vi "5_VNA_KEYSIGHT_T1_measurements_(Subprog_Rabi).vi"(0 "VNA Power dBm":dbl=5.0 caption="VNA Power, dBm" format="%#.3f", 1 "Center Freq:":dbl=6954420000.0 format="%^#.6e", 2 "Span Freq:":dbl=10000.0 format="%^#.3e", 3 "Bandwidth:":dbl=10.0 caption="Bandwidth (1 to 1e6 Hz):" format="%#.3f", 4 "Sweep Type":i32(ring)=4 caption="Sweep Type:" items=["Lin. Frequency", "Log. Frequency", "Segmented Frequency", "Power", "CW Mode", "Time"], 5 "Points:":i32=4, 6 "File name":string="C:\\ExperimentBlue\\Photon_Source_Dec8'17\\Photon_Source_Dec8'17_Q_osc_05CAL", 7 "Comments":string=" cell Ay\nI=0.0082mA \nf=6.93602GHz\nPulse length sweep 1.5 to 51.5 ns 251 points\nPower  10 to -15 dBm 5 points \nKeysight frequency of pulse generator 10MHz ( 100ns pulse to pulse) \nbandwidth 5Hz\nTransmission Input (VNA):  -chopper1-20-40(4K)\nOut: ~+35dB(4K)+35(RT)", 8 "Dt0 (ns)":dbl=2.0, 9 "Dt1 (ns)":dbl=52.0, 10 "Numeric":u32=251, 11 "save":bool, 12 "Gen Power dBm 2":dbl caption="Gen Power, dBm" format="%#.3f", 13 "Gen Freq:":dbl=10905300000.0 format="%^#.6e") -> (14 "ampl":dbl[](graph)=[-5.350595642994449e-06, -5.748102353209106e-06, -6.142002803244395e-06, -7.127714638954787e-06, -7.280243835339206e-06, -7.58689486701769e-06, -7.235651878545468e-06, -7.886853154559503e-06, -8.111406259558862e-06, -8.24788344289118e-06, -7.998179626156343e-06, -8.358461400348462e-06, -8.104447488221922e-06, -8.498929219058482e-06, -8.536551149518347e-06, -8.1918499290623e-06, -8.209974566852907e-06, -8.195522696041735e-06, -8.220921131396608e-06, -7.921980113678728e-06, -7.674006610614015e-06, -7.494857754863916e-06, -7.402117944366182e-06, -6.798555773457339e-06, -7.21594403785275e-06, -7.021225655989839e-06, -6.167525157252384e-06, -5.991822149553627e-06, -5.853642846886942e-06, -5.251931042948854e-06, -5.243861437520537e-06, -4.8519466417928925e-06, -4.460138825379545e-06, -3.7825817003067637e-06, -3.2926087101259327e-06, -2.9916130301899106e-06, -2.481511216956278e-06, -2.7349177571522887e-06, -1.8771629584080074e-06, -1.5279611602636578e-06, -1.2175324712870859e-06, -5.379010161732367e-07, 6.21079596641039e-08, 8.855542699137692e-08, 4.6134938713748847e-07, 9.043904896088861e-07, 1.3269203407162422e-06, 1.5433369071615743e-06, 1.8643518728822528e-06, 2.399540846909076e-06, 2.143343635907513e-06, 3.011504986716318e-06, 2.7575520675782172e-06, 3.1280499115382554e-06, 3.4887555671048176e-06, 3.906060385361343e-06, 3.6936039009560773e-06, 4.253995143699285e-06, 4.361229116511822e-06, 4.483709631131205e-06, 4.3406083705122e-06, 4.7702748133815476e-06, 5.171184739083401e-06, 4.7876910684863105e-06, 5.051228299635113e-06, 5.085999646325945e-06, 5.146128160049557e-06, 4.943444650962192e-06, 4.87218039779691e-06, 4.565880658446986e-06, 4.918219360661169e-06, 4.184556587460975e-06, 4.655326165448059e-06, 4.499653073253285e-06, 4.171141711140081e-06, 3.84760699034814e-06, 3.771454544221342e-06, 3.763502945730579e-06, 2.8933102385053644e-06, 2.874121037166333e-06, 2.9050245302641997e-06, 2.5922465169969655e-06, 2.1929668321263307e-06, 2.0736858346026565e-06, 1.7167542409879388e-06, 1.4624756374814751e-06, 7.380953093161227e-07, 6.440802060581063e-07, 5.810447483156622e-07, 1.042342834267628e-07, -1.5370875949827212e-07, -5.226669990143761e-07, -7.853622037146126e-07, -1.1198991956007376e-06, -1.5348909698786885e-06, -1.9866505738264095e-06, -1.855540432416092e-06, -2.205690805112681e-06, -2.46238369072671e-06, -2.5284312528128794e-06, -3.0026736226318454e-06, -3.084425941324298e-06, -3.5802571005660857e-06, -3.7021916341473124e-06, -3.686246998313437e-06, -3.4973670040017173e-06, -3.839401415461907e-06, -4.0807350387694905e-06, -4.076152492871189e-06, -4.00435214942263e-06, -4.185059196970542e-06, -4.610368591784209e-06, -4.490104402066208e-06, -4.114603484595135e-06, -4.458382022676233e-06, -4.066545898240292e-06, -3.910781515514827e-06, -4.353571966930759e-06, -3.840349222627992e-06, -3.952571830723173e-06, -3.831163269296667e-06, -3.859261880734265e-06, -3.651557278772088e-06, -3.3495256275273273e-06, -3.446964456088609e-06, -3.3059969837268004e-06, -3.199198999936925e-06, -2.674532879609615e-06, -2.8501009978754155e-06, -2.359338509450027e-06, -2.564694455031713e-06, -2.4649946226418255e-06, -1.9019816477339193e-06, -2.14103451412484e-06, -1.5622521800651155e-06, -1.6103490736441017e-06, -1.6571096637107987e-06, -1.1951571394774874e-06, -1.145164489457784e-06, -9.099043580818036e-07, -4.058469613710259e-07, -5.379223795287658e-07, -3.0455108035454254e-07, -2.0577362391804844e-07, 1.5127773167478138e-07, 3.7407837538694356e-07, 3.06401084060326e-07, 5.40101289914219e-07, 4.2760392915397455e-07, 8.288863710959048e-07, 6.351086767608649e-07, 7.104995063400566e-07, 1.0201038023183173e-06, 1.287821618234375e-06, 1.2846170278635327e-06, 1.1899174978680094e-06, 1.5496536889259005e-06, 1.7193417818361922e-06, 1.2724093494398403e-06, 1.5057571260967961e-06, 1.9633712611266674e-06, 1.5103734369859012e-06, 1.6298976390771713e-06, 1.6734024086417776e-06, 1.480321373037441e-06, 1.6955580974808981e-06, 1.634662169180956e-06, 1.5839247566873382e-06, 1.6462490464164148e-06, 1.4869986841858918e-06, 1.1734323663858959e-06, 1.4257581142373965e-06, 9.750721545742635e-07, 9.460953975803934e-07, 8.49423898330315e-07, 9.841615025152353e-07, 3.2011315020952246e-07, 6.019439595661424e-07, 3.982507532640514e-07, 5.402164049428264e-09, 2.1368394520493444e-07, -3.2420262030541264e-09, -2.370501128723403e-08, -3.75823718812285e-07, -5.397894007330705e-07, -6.145908812982271e-07, -7.628222959965569e-07, -1.1389743690415342e-06, -1.3418293747236025e-06, -1.3894015182813746e-06, -1.369024602126956e-06, -1.6103733457839553e-06, -1.764732246556377e-06, -1.770231932596289e-06, -2.033277155533142e-06, -2.006639647333941e-06, -1.9775290240886534e-06, -1.9851460990594205e-06, -2.3815686063244353e-06, -2.5377885322086513e-06, -2.6544240085968345e-06, -2.5942898105313365e-06, -2.5383228035025236e-06, -3.001205584496347e-06, -2.8813012136197362e-06, -2.361626343372336e-06, -2.9243871040307567e-06, -2.813621961195168e-06, -2.776986320895958e-06, -2.75323276355266e-06, -2.9784823709633193e-06, -2.7528085979611205e-06, -2.9853597993678704e-06, -2.6832433377421694e-06, -2.706799818952277e-06, -2.6102525794158282e-06, -2.5532914378345595e-06, -2.4495236345956073e-06, -2.8292968750065475e-06, -2.7355002885087742e-06, -2.578310500211955e-06, -2.295727739465292e-06, -2.2412349949263444e-06, -2.179298746796121e-06, -2.216602865701134e-06, -2.0977130361643503e-06, -2.037876214444623e-06, -2.1244423464850115e-06, -1.7360226820528626e-06, -1.8201646980742221e-06, -1.7183827480948821e-06, -1.7188583854022004e-06, -1.6155918274307621e-06, -1.6261506914361235e-06, -1.5005421118985398e-06, -1.3091014494648334e-06, -1.3107754170960109e-06, -1.1031796702809515e-06, -1.0116501982793125e-06, -1.0896207669475189e-06, -1.2497122128252158e-06, -9.131707017218105e-07, -8.035339078560353e-07, -7.777753410209698e-07, -8.975365659580346e-07, -8.154549675509772e-07, -7.933004440019431e-07, -4.751387692181199e-07, -4.0351462438081864e-07, -7.113754421084194e-07, -4.4958940748074394e-07], 19 "phase":dbl[](graph)=[-7.019170425337506e-06, -7.572992899440578e-06, -8.083594366325997e-06, -8.282980843432597e-06, -9.005763786262833e-06, -9.200682825394324e-06, -9.523038443148835e-06, -9.838679261520156e-06, -1.0108198466696194e-05, -1.0165816092921887e-05, -1.029021063914115e-05, -1.031981514643121e-05, -1.0695643595681759e-05, -1.0575919532129774e-05, -1.088692602024821e-05, -1.0727918834163575e-05, -1.0352908930144622e-05, -1.0479309594302322e-05, -1.026801805892319e-05, -1.0114804808836197e-05, -9.96231437966344e-06, -1.0128693247679621e-05, -9.729141083880677e-06, -9.54572783484764e-06, -9.351148946734611e-06, -8.996363249025308e-06, -8.951605195761658e-06, -8.266448276117444e-06, -8.23883738121367e-06, -7.827569334040163e-06, -7.317791073546687e-06, -6.8893916704837466e-06, -6.896793706800963e-06, -6.259986207624024e-06, -6.152467562969832e-06, -5.733801913265779e-06, -5.14998862399807e-06, -5.054679149907315e-06, -4.6699628910573665e-06, -4.385781835480884e-06, -3.852076304156071e-06, -3.4347103223808517e-06, -3.1505589390690147e-06, -2.882839055473596e-06, -2.4267251319542993e-06, -2.0543377274861996e-06, -1.8744106853318954e-06, -1.8350467883010424e-06, -1.1185632899923803e-06, -1.2640456645840459e-06, -7.661341072662253e-07, -5.049992815031602e-07, -3.6385645785230736e-07, -4.366051165050068e-08, 3.774253407584638e-07, 5.211261182580529e-07, 4.2912330577848934e-07, 8.784667500094656e-07, 7.522494485101561e-07, 8.956429340400973e-07, 9.095790503010903e-07, 1.184701375223085e-06, 9.438186765464707e-07, 1.0257956688519698e-06, 1.3411245447514375e-06, 1.0582824359062215e-06, 1.352960623535182e-06, 1.153802429598727e-06, 9.581724071949793e-07, 7.940060662292581e-07, 7.361063865118922e-07, 9.280784922793828e-07, 6.255717437397834e-07, 2.950829518511e-07, 5.000459566417703e-07, -2.9220700525911525e-07, -1.555246562645607e-07, -7.036747007305166e-07, -9.239828386853333e-07, -8.351137665840724e-07, -1.3118549304635962e-06, -1.7194672636833275e-06, -1.8967983805850963e-06, -2.3815821350581245e-06, -2.2676868240978365e-06, -3.2337324000764056e-06, -3.3083579751291836e-06, -3.5524304280443175e-06, -3.800510512519395e-06, -3.80134156330314e-06, -4.356420959084062e-06, -4.827017278330459e-06, -5.025575205763744e-06, -5.325945721779135e-06, -5.358401494959253e-06, -6.143812811387761e-06, -6.290685405474505e-06, -6.308485922090767e-06, -6.2665590121468995e-06, -6.645629355261917e-06, -6.524124955831212e-06, -6.957865366530314e-06, -6.78449987390195e-06, -7.311455647140974e-06, -7.419965868393774e-06, -7.837340831429174e-06, -7.111336913112609e-06, -7.561965958302607e-06, -7.808766213202034e-06, -7.69942892020481e-06, -7.712463570896944e-06, -7.581047043458965e-06, -8.152239843184361e-06, -7.779721727274591e-06, -7.729709182058286e-06, -7.868625402807083e-06, -7.543547440036491e-06, -7.2425145845045336e-06, -7.3920455179177225e-06, -7.1634891583016724e-06, -7.435683642142976e-06, -7.109604098332056e-06, -7.161242933761969e-06, -6.776788495699293e-06, -7.035438557068119e-06, -6.850255317658593e-06, -6.483218953690084e-06, -6.188151473907055e-06, -6.034766897755617e-06, -6.058859753466095e-06, -5.548203489524894e-06, -5.673710234077589e-06, -5.174108423489088e-06, -5.141609562997473e-06, -5.159966576684383e-06, -4.946431545249652e-06, -4.847265131502354e-06, -4.7356253389807534e-06, -4.414978661770874e-06, -4.251912287145387e-06, -3.852206191368168e-06, -4.0920668311628106e-06, -3.608850192904356e-06, -3.4423123906890396e-06, -3.716679202625528e-06, -3.326873752484971e-06, -3.0694831139044254e-06, -3.3468560332039488e-06, -3.054596163565293e-06, -2.8194069727760507e-06, -2.8818586770285037e-06, -2.564631074619683e-06, -2.6920887421510997e-06, -2.6940328439195582e-06, -2.4095087098885415e-06, -2.3805068849469535e-06, -2.5056550043700554e-06, -2.443875587232469e-06, -2.177272733661084e-06, -2.4558263476137654e-06, -2.4497868480466423e-06, -2.4176401893782895e-06, -2.682157230537996e-06, -2.536869828873023e-06, -2.40958911490452e-06, -2.6013264005086967e-06, -2.5794037696869054e-06, -3.0161366453285154e-06, -2.6545178002379544e-06, -2.945309233837179e-06, -3.0584037062908465e-06, -3.5290661344333785e-06, -3.1222189136315137e-06, -3.4254662750754505e-06, -3.7309258118511934e-06, -3.883167721596692e-06, -3.7888983683842525e-06, -3.7286271776793e-06, -4.267222948328708e-06, -4.215672788632219e-06, -4.799514613296196e-06, -4.049223491620069e-06, -4.806045012628601e-06, -4.765840685649891e-06, -4.712963459496677e-06, -4.8368552825195366e-06, -5.012265887671674e-06, -5.605749834103335e-06, -5.384020710152981e-06, -5.640716835841886e-06, -5.535724994842894e-06, -5.903570922782819e-06, -5.744383543060394e-06, -6.076711542846169e-06, -5.908389880460163e-06, -6.2967959593152045e-06, -6.162372528706328e-06, -6.263441719056573e-06, -6.3702756278871675e-06, -6.32096828212525e-06, -6.562064413628832e-06, -6.547394150402397e-06, -6.580206786566123e-06, -6.6398285980540095e-06, -6.828778737144603e-06, -6.4207348486888804e-06, -6.490270152426092e-06, -6.515018526442873e-06, -6.581525326510018e-06, -6.594809974558302e-06, -6.453879677792429e-06, -6.79197262343223e-06, -6.798417985010019e-06, -6.491771046057693e-06, -6.526720881083747e-06, -6.384674179571448e-06, -6.509471973004111e-06, -6.414986501113162e-06, -6.234956458683882e-06, -6.2904579181122244e-06, -6.238534183466982e-06, -6.273923645494506e-06, -5.890055604140798e-06, -6.004691272210039e-06, -5.961678311905416e-06, -5.60485193545901e-06, -5.890900865779258e-06, -5.728247288061539e-06, -5.71459065668023e-06, -5.6967975297084195e-06, -5.555835969062173e-06, -5.256393819763616e-06, -5.2477131475825445e-06, -5.247593207968748e-06, -5.350767878553597e-06, -5.333628905646037e-06, -5.198694452701602e-06, -4.963535388924356e-06, -5.009527740185149e-06, -4.453745532373432e-06, -4.926283281747601e-06, -4.547008074951009e-06, -4.7042154847076745e-06, -4.747226967083407e-06, -4.635495542970602e-06, -4.49793731149839e-06, -4.559130957204616e-06, -4.701467787526781e-06, -4.702796445599233e-06, -4.415612238517497e-06, -4.52840652087616e-06])   [LabVIEW 2013]
uses:
  <vilib>/Analysis/NI_AALBase.lvlib
  <vilib>/Analysis/baseanly.llb/Mean (DBL).vi
  <instrlib>/Rohde&Schwarz Vector Network Analyzer/Rohde&Schwarz Vector Network Analyzer.lvlib
panel:
  in  "Ring":u16(ring) items=["Pulse Shift Calibration", "T1 measurement"]
  out "Waveform Graph 2":dbl[](graph)=[-2.2221124422202494, -2.2200494150598864, -2.22054687555374, -2.2813692262672824, -2.2506372258925262, -2.26035908210725, -2.2205431360999093, -2.2465225043911956, -2.247034345801779, -2.252410802151737, -2.2315174356881977, -2.251570699160605, -2.219228532735236, -2.247735449942519, -2.2357730706088486, -2.2229454228604424, -2.241261362587479, -2.234506489472927, -2.245923542606182, -2.235213072381829, -2.2271656113017997, -2.2078427166064345, -2.221185880687629, -2.1896695136273903, -2.2280187758346655, -2.233503304957881, -2.1740916174174107, -2.1979972395375613, -2.1885304421115324, -2.1617605168228144, -2.1925704607839447, -2.1843779293512475, -2.1448463827428856, -2.1143332172734173, -2.0621815638276297, -2.0516924087743607, -2.0198170903435035, -2.066754972840862, -1.9529957650207677, -1.9060358490862137, -1.8769318504176142, -1.726141921489059, -1.551085565186052, -1.5400878525067452, -1.3829263568713952, -1.1560929446483101, -0.9547791124266966, -0.8715305192592462, -0.5404006345918181, -0.4848464421487932, -0.34329462610936456, -0.16614419088094917, -0.13119121203076994, -0.013956835064683466, 0.10776426448886352, 0.13263153817421908, 0.11566157655036537, 0.20364145310501736, 0.17080499526778212, 0.19715986817145928, 0.20656216976967054, 0.24342583588988514, 0.18052791711975594, 0.2110657483169402, 0.2595171973551559, 0.20515025024512784, 0.2570904199282286, 0.22929562642177953, 0.1941838278195652, 0.17217803058580022, 0.14856649652833964, 0.21825376571269267, 0.13357745712488828, 0.06548527695229357, 0.11931287033258386, -0.07579962255318175, -0.04121396317718357, -0.18483912418150655, -0.30911453237721853, -0.2827768403838537, -0.4241682085492582, -0.5856762880987345, -0.7131073752889852, -0.8543968263078259, -0.9227979241818781, -1.1460676995353924, -1.3512908802483115, -1.3914377765807178, -1.419085113448628, -1.5433828019515092, -1.6060649622360101, -1.6786556026742614, -1.7258156155951736, -1.7780493664571155, -1.8497720515141458, -1.8835423107580829, -1.8576287081929448, -1.9071492374579924, -1.9452019952135486, -1.9343498475916896, -2.0021344441342155, -1.9880650878931068, -2.0563664069434715, -2.0395149482186863, -2.0318815202783984, -1.990522446503196, -2.0658511419319145, -2.065650386834191, -2.0518862750216837, -2.0503819785658073, -2.067968101516807, -2.1171825838775367, -2.0742394821005004, -2.0572865701670437, -2.0939712129344246, -2.0477974698596264, -2.049076926431744, -2.1120340406068565, -2.049941304549976, -2.074994602403109, -2.0465616437371685, -2.068113242334879, -2.0423369110411205, -2.0298449758096195, -2.0263660817750417, -2.020434841824136, -2.029196992794578, -1.978751479362645, -2.0120232234838236, -1.9421341611880314, -2.003796081836927, -1.9806514965134467, -1.923060086421989, -1.9653715255507558, -1.8647869786316142, -1.8855325996641679, -1.9002055120394206, -1.8180097653312641, -1.824585110222654, -1.7816153777828392, -1.6757635298129716, -1.7015018190888993, -1.6549869043375756, -1.6305030072196787, -1.5301163900716812, -1.4588252225530398, -1.4713041922306656, -1.4107999761308114, -1.431713078921382, -1.284859462699359, -1.3538820510403298, -1.3005366667363418, -1.2085876850018074, -1.1248807725031937, -1.0809857977123978, -1.1072616226786955, -1.0169119447770274, -0.9577046170580744, -1.041922570804954, -1.0207734830165345, -0.8951744503606424, -1.0123908705644693, -1.0247477161996408, -0.9876791829403154, -1.0198950424763618, -0.9931531132853096, -1.0059392786561479, -1.087231587819844, -1.015678698276403, -1.1032602007634085, -1.2044421445787075, -1.1868426866585982, -1.2680927449116148, -1.3013198155159527, -1.3469409737242553, -1.3225798696208182, -1.4865093650461314, -1.4107387915976213, -1.4777380317239253, -1.5695148798317882, -1.5263037183873518, -1.5715969804305876, -1.5757286191468585, -1.649491275031389, -1.6848323318110747, -1.6971831913424815, -1.7218284748673327, -1.7712473782272706, -1.8150448879730567, -1.8123051545733142, -1.8132389806596525, -1.837097021722014, -1.8688546324376627, -1.8542655068601206, -1.9022356789843693, -1.8792980678558984, -1.8813189423639314, -1.8777226273574936, -1.928564052446991, -1.9525842070365895, -1.9551850148775656, -1.94805057408691, -1.9389592497479615, -1.9953125916293035, -1.9700680868198772, -1.9232507592064303, -1.9941326276753457, -1.9784690362549648, -1.9700693755267644, -1.9662843310264109, -2.0031745533339986, -1.9558660968106016, -1.9845704436945957, -1.962740954169606, -1.9639325880875806, -1.9588923567604022, -1.9445973510447443, -1.9355536099748598, -1.9967890317788455, -1.9809929986786614, -1.9627050215137167, -1.9215790726286834, -1.9343903833346052, -1.9189456958370024, -1.926766066796904, -1.9289245120909744, -1.9038463108288426, -1.9259423843913106, -1.8657244955094845, -1.8800516842623896, -1.8707571123101403, -1.8868391186030182, -1.8694538115127195, -1.8712971229669364, -1.8442082768353885, -1.8114813953939026, -1.817783858710915, -1.7894982571991789, -1.7700615920931608, -1.8107359177553446, -1.819237925501068, -1.7689887938445552, -1.7399750440670247, -1.733191361488536, -1.7620522908712142, -1.7501436462206248, -1.7430740255534625, -1.671516149616777, -1.6563898097010057, -1.7305284307855928, -1.6697540708562737]
  out "No of Values":i32
  in  "Boolean":bool
  out "Pow":dbl=34.32006687269598
  out "Waveform Graph":dbl[][](graph)=[[-5.350595642994449e-06, -5.748102353209106e-06, -6.142002803244395e-06, -7.127714638954787e-06, -7.280243835339206e-06, -7.58689486701769e-06, -7.235651878545468e-06, -7.886853154559503e-06, -8.111406259558862e-06, -8.24788344289118e-06, -7.998179626156343e-06, -8.358461400348462e-06, -8.104447488221922e-06, -8.498929219058482e-06, -8.536551149518347e-06, -8.1918499290623e-06, -8.209974566852907e-06, -8.195522696041735e-06, -8.220921131396608e-06, -7.921980113678728e-06, -7.674006610614015e-06, -7.494857754863916e-06, -7.402117944366182e-06, -6.798555773457339e-06, -7.21594403785275e-06, -7.021225655989839e-06, -6.167525157252384e-06, -5.991822149553627e-06, -5.853642846886942e-06, -5.251931042948854e-06, -5.243861437520537e-06, -4.8519466417928925e-06, -4.460138825379545e-06, -3.7825817003067637e-06, -3.2926087101259327e-06, -2.9916130301899106e-06, -2.481511216956278e-06, -2.7349177571522887e-06, -1.8771629584080074e-06, -1.5279611602636578e-06, -1.2175324712870859e-06, -5.379010161732367e-07, 6.21079596641039e-08, 8.855542699137692e-08, 4.6134938713748847e-07, 9.043904896088861e-07, 1.3269203407162422e-06, 1.5433369071615743e-06, 1.8643518728822528e-06, 2.399540846909076e-06, 2.143343635907513e-06, 3.011504986716318e-06, 2.7575520675782172e-06, 3.1280499115382554e-06, 3.4887555671048176e-06, 3.906060385361343e-06, 3.6936039009560773e-06, 4.253995143699285e-06, 4.361229116511822e-06, 4.483709631131205e-06, 4.3406083705122e-06, 4.7702748133815476e-06, 5.171184739083401e-06, 4.7876910684863105e-06, 5.051228299635113e-06, 5.085999646325945e-06, 5.146128160049557e-06, 4.943444650962192e-06, 4.87218039779691e-06, 4.565880658446986e-06, 4.918219360661169e-06, 4.184556587460975e-06, 4.655326165448059e-06, 4.499653073253285e-06, 4.171141711140081e-06, 3.84760699034814e-06, 3.771454544221342e-06, 3.763502945730579e-06, 2.8933102385053644e-06, 2.874121037166333e-06, 2.9050245302641997e-06, 2.5922465169969655e-06, 2.1929668321263307e-06, 2.0736858346026565e-06, 1.7167542409879388e-06, 1.4624756374814751e-06, 7.380953093161227e-07, 6.440802060581063e-07, 5.810447483156622e-07, 1.042342834267628e-07, -1.5370875949827212e-07, -5.226669990143761e-07, -7.853622037146126e-07, -1.1198991956007376e-06, -1.5348909698786885e-06, -1.9866505738264095e-06, -1.855540432416092e-06, -2.205690805112681e-06, -2.46238369072671e-06, -2.5284312528128794e-06, -3.0026736226318454e-06, -3.084425941324298e-06, -3.5802571005660857e-06, -3.7021916341473124e-06, -3.686246998313437e-06, -3.4973670040017173e-06, -3.839401415461907e-06, -4.0807350387694905e-06, -4.076152492871189e-06, -4.00435214942263e-06, -4.185059196970542e-06, -4.610368591784209e-06, -4.490104402066208e-06, -4.114603484595135e-06, -4.458382022676233e-06, -4.066545898240292e-06, -3.910781515514827e-06, -4.353571966930759e-06, -3.840349222627992e-06, -3.952571830723173e-06, -3.831163269296667e-06, -3.859261880734265e-06, -3.651557278772088e-06, -3.3495256275273273e-06, -3.446964456088609e-06, -3.3059969837268004e-06, -3.199198999936925e-06, -2.674532879609615e-06, -2.8501009978754155e-06, -2.359338509450027e-06, -2.564694455031713e-06, -2.4649946226418255e-06, -1.9019816477339193e-06, -2.14103451412484e-06, -1.5622521800651155e-06, -1.6103490736441017e-06, -1.6571096637107987e-06, -1.1951571394774874e-06, -1.145164489457784e-06, -9.099043580818036e-07, -4.058469613710259e-07, -5.379223795287658e-07, -3.0455108035454254e-07, -2.0577362391804844e-07, 1.5127773167478138e-07, 3.7407837538694356e-07, 3.06401084060326e-07, 5.40101289914219e-07, 4.2760392915397455e-07, 8.288863710959048e-07, 6.351086767608649e-07, 7.104995063400566e-07, 1.0201038023183173e-06, 1.287821618234375e-06, 1.2846170278635327e-06, 1.1899174978680094e-06, 1.5496536889259005e-06, 1.7193417818361922e-06, 1.2724093494398403e-06, 1.5057571260967961e-06, 1.9633712611266674e-06, 1.5103734369859012e-06, 1.6298976390771713e-06, 1.6734024086417776e-06, 1.480321373037441e-06, 1.6955580974808981e-06, 1.634662169180956e-06, 1.5839247566873382e-06, 1.6462490464164148e-06, 1.4869986841858918e-06, 1.1734323663858959e-06, 1.4257581142373965e-06, 9.750721545742635e-07, 9.460953975803934e-07, 8.49423898330315e-07, 9.841615025152353e-07, 3.2011315020952246e-07, 6.019439595661424e-07, 3.982507532640514e-07, 5.402164049428264e-09, 2.1368394520493444e-07, -3.2420262030541264e-09, -2.370501128723403e-08, -3.75823718812285e-07, -5.397894007330705e-07, -6.145908812982271e-07, -7.628222959965569e-07, -1.1389743690415342e-06, -1.3418293747236025e-06, -1.3894015182813746e-06, -1.369024602126956e-06, -1.6103733457839553e-06, -1.764732246556377e-06, -1.770231932596289e-06, -2.033277155533142e-06, -2.006639647333941e-06, -1.9775290240886534e-06, -1.9851460990594205e-06, -2.3815686063244353e-06, -2.5377885322086513e-06, -2.6544240085968345e-06, -2.5942898105313365e-06, -2.5383228035025236e-06, -3.001205584496347e-06, -2.8813012136197362e-06, -2.361626343372336e-06, -2.9243871040307567e-06, -2.813621961195168e-06, -2.776986320895958e-06, -2.75323276355266e-06, -2.9784823709633193e-06, -2.7528085979611205e-06, -2.9853597993678704e-06, -2.6832433377421694e-06, -2.706799818952277e-06, -2.6102525794158282e-06, -2.5532914378345595e-06, -2.4495236345956073e-06, -2.8292968750065475e-06, -2.7355002885087742e-06, -2.578310500211955e-06, -2.295727739465292e-06, -2.2412349949263444e-06, -2.179298746796121e-06, -2.216602865701134e-06, -2.0977130361643503e-06, -2.037876214444623e-06, -2.1244423464850115e-06, -1.7360226820528626e-06, -1.8201646980742221e-06, -1.7183827480948821e-06, -1.7188583854022004e-06, -1.6155918274307621e-06, -1.6261506914361235e-06, -1.5005421118985398e-06, -1.3091014494648334e-06, -1.3107754170960109e-06, -1.1031796702809515e-06, -1.0116501982793125e-06, -1.0896207669475189e-06, -1.2497122128252158e-06, -9.131707017218105e-07, -8.035339078560353e-07, -7.777753410209698e-07, -8.975365659580346e-07, -8.154549675509772e-07, -7.933004440019431e-07, -4.751387692181199e-07, -4.0351462438081864e-07, -7.113754421084194e-07, -4.4958940748074394e-07], [-7.019170425337506e-06, -7.572992899440578e-06, -8.083594366325997e-06, -8.282980843432597e-06, -9.005763786262833e-06, -9.200682825394324e-06, -9.523038443148835e-06, -9.838679261520156e-06, -1.0108198466696194e-05, -1.0165816092921887e-05, -1.029021063914115e-05, -1.031981514643121e-05, -1.0695643595681759e-05, -1.0575919532129774e-05, -1.088692602024821e-05, -1.0727918834163575e-05, -1.0352908930144622e-05, -1.0479309594302322e-05, -1.026801805892319e-05, -1.0114804808836197e-05, -9.96231437966344e-06, -1.0128693247679621e-05, -9.729141083880677e-06, -9.54572783484764e-06, -9.351148946734611e-06, -8.996363249025308e-06, -8.951605195761658e-06, -8.266448276117444e-06, -8.23883738121367e-06, -7.827569334040163e-06, -7.317791073546687e-06, -6.8893916704837466e-06, -6.896793706800963e-06, -6.259986207624024e-06, -6.152467562969832e-06, -5.733801913265779e-06, -5.14998862399807e-06, -5.054679149907315e-06, -4.6699628910573665e-06, -4.385781835480884e-06, -3.852076304156071e-06, -3.4347103223808517e-06, -3.1505589390690147e-06, -2.882839055473596e-06, -2.4267251319542993e-06, -2.0543377274861996e-06, -1.8744106853318954e-06, -1.8350467883010424e-06, -1.1185632899923803e-06, -1.2640456645840459e-06, -7.661341072662253e-07, -5.049992815031602e-07, -3.6385645785230736e-07, -4.366051165050068e-08, 3.774253407584638e-07, 5.211261182580529e-07, 4.2912330577848934e-07, 8.784667500094656e-07, 7.522494485101561e-07, 8.956429340400973e-07, 9.095790503010903e-07, 1.184701375223085e-06, 9.438186765464707e-07, 1.0257956688519698e-06, 1.3411245447514375e-06, 1.0582824359062215e-06, 1.352960623535182e-06, 1.153802429598727e-06, 9.581724071949793e-07, 7.940060662292581e-07, 7.361063865118922e-07, 9.280784922793828e-07, 6.255717437397834e-07, 2.950829518511e-07, 5.000459566417703e-07, -2.9220700525911525e-07, -1.555246562645607e-07, -7.036747007305166e-07, -9.239828386853333e-07, -8.351137665840724e-07, -1.3118549304635962e-06, -1.7194672636833275e-06, -1.8967983805850963e-06, -2.3815821350581245e-06, -2.2676868240978365e-06, -3.2337324000764056e-06, -3.3083579751291836e-06, -3.5524304280443175e-06, -3.800510512519395e-06, -3.80134156330314e-06, -4.356420959084062e-06, -4.827017278330459e-06, -5.025575205763744e-06, -5.325945721779135e-06, -5.358401494959253e-06, -6.143812811387761e-06, -6.290685405474505e-06, -6.308485922090767e-06, -6.2665590121468995e-06, -6.645629355261917e-06, -6.524124955831212e-06, -6.957865366530314e-06, -6.78449987390195e-06, -7.311455647140974e-06, -7.419965868393774e-06, -7.837340831429174e-06, -7.111336913112609e-06, -7.561965958302607e-06, -7.808766213202034e-06, -7.69942892020481e-06, -7.712463570896944e-06, -7.581047043458965e-06, -8.152239843184361e-06, -7.779721727274591e-06, -7.729709182058286e-06, -7.868625402807083e-06, -7.543547440036491e-06, -7.2425145845045336e-06, -7.3920455179177225e-06, -7.1634891583016724e-06, -7.435683642142976e-06, -7.109604098332056e-06, -7.161242933761969e-06, -6.776788495699293e-06, -7.035438557068119e-06, -6.850255317658593e-06, -6.483218953690084e-06, -6.188151473907055e-06, -6.034766897755617e-06, -6.058859753466095e-06, -5.548203489524894e-06, -5.673710234077589e-06, -5.174108423489088e-06, -5.141609562997473e-06, -5.159966576684383e-06, -4.946431545249652e-06, -4.847265131502354e-06, -4.7356253389807534e-06, -4.414978661770874e-06, -4.251912287145387e-06, -3.852206191368168e-06, -4.0920668311628106e-06, -3.608850192904356e-06, -3.4423123906890396e-06, -3.716679202625528e-06, -3.326873752484971e-06, -3.0694831139044254e-06, -3.3468560332039488e-06, -3.054596163565293e-06, -2.8194069727760507e-06, -2.8818586770285037e-06, -2.564631074619683e-06, -2.6920887421510997e-06, -2.6940328439195582e-06, -2.4095087098885415e-06, -2.3805068849469535e-06, -2.5056550043700554e-06, -2.443875587232469e-06, -2.177272733661084e-06, -2.4558263476137654e-06, -2.4497868480466423e-06, -2.4176401893782895e-06, -2.682157230537996e-06, -2.536869828873023e-06, -2.40958911490452e-06, -2.6013264005086967e-06, -2.5794037696869054e-06, -3.0161366453285154e-06, -2.6545178002379544e-06, -2.945309233837179e-06, -3.0584037062908465e-06, -3.5290661344333785e-06, -3.1222189136315137e-06, -3.4254662750754505e-06, -3.7309258118511934e-06, -3.883167721596692e-06, -3.7888983683842525e-06, -3.7286271776793e-06, -4.267222948328708e-06, -4.215672788632219e-06, -4.799514613296196e-06, -4.049223491620069e-06, -4.806045012628601e-06, -4.765840685649891e-06, -4.712963459496677e-06, -4.8368552825195366e-06, -5.012265887671674e-06, -5.605749834103335e-06, -5.384020710152981e-06, -5.640716835841886e-06, -5.535724994842894e-06, -5.903570922782819e-06, -5.744383543060394e-06, -6.076711542846169e-06, -5.908389880460163e-06, -6.2967959593152045e-06, -6.162372528706328e-06, -6.263441719056573e-06, -6.3702756278871675e-06, -6.32096828212525e-06, -6.562064413628832e-06, -6.547394150402397e-06, -6.580206786566123e-06, -6.6398285980540095e-06, -6.828778737144603e-06, -6.4207348486888804e-06, -6.490270152426092e-06, -6.515018526442873e-06, -6.581525326510018e-06, -6.594809974558302e-06, -6.453879677792429e-06, -6.79197262343223e-06, -6.798417985010019e-06, -6.491771046057693e-06, -6.526720881083747e-06, -6.384674179571448e-06, -6.509471973004111e-06, -6.414986501113162e-06, -6.234956458683882e-06, -6.2904579181122244e-06, -6.238534183466982e-06, -6.273923645494506e-06, -5.890055604140798e-06, -6.004691272210039e-06, -5.961678311905416e-06, -5.60485193545901e-06, -5.890900865779258e-06, -5.728247288061539e-06, -5.71459065668023e-06, -5.6967975297084195e-06, -5.555835969062173e-06, -5.256393819763616e-06, -5.2477131475825445e-06, -5.247593207968748e-06, -5.350767878553597e-06, -5.333628905646037e-06, -5.198694452701602e-06, -4.963535388924356e-06, -5.009527740185149e-06, -4.453745532373432e-06, -4.926283281747601e-06, -4.547008074951009e-06, -4.7042154847076745e-06, -4.747226967083407e-06, -4.635495542970602e-06, -4.49793731149839e-06, -4.559130957204616e-06, -4.701467787526781e-06, -4.702796445599233e-06, -4.415612238517497e-06, -4.52840652087616e-06], [8.825963244584914e-06, 9.507413008697238e-06, 1.0152275425458049e-05, 1.0927583796386178e-05, 1.1580402915095726e-05, 1.1925331784763283e-05, 1.1960055154437589e-05, 1.2609601987876223e-05, 1.2960346744965197e-05, 1.3090889890401954e-05, 1.303300856786936e-05, 1.328015292222293e-05, 1.341934651967803e-05, 1.3567677465972209e-05, 1.3834661676336742e-05, 1.3497949761822333e-05, 1.3213114913003665e-05, 1.33034778097523e-05, 1.3153544735432195e-05, 1.2847842046132771e-05, 1.257529662707789e-05, 1.260013173229687e-05, 1.222487367183656e-05, 1.1719269623222905e-05, 1.1811597477963701e-05, 1.1411930661406207e-05, 1.087058425964898e-05, 1.0209608208624193e-05, 1.0106610508622285e-05, 9.426219887054185e-06, 9.002674545488942e-06, 8.426452622790693e-06, 8.213318560474043e-06, 7.314051656854676e-06, 6.978117886034393e-06, 6.4673203804181816e-06, 5.71666692638196e-06, 5.747134629264799e-06, 5.033119726002152e-06, 4.644324236711767e-06, 4.039910540058918e-06, 3.4765748232807784e-06, 3.15117105648064e-06, 2.88419886336111e-06, 2.4701898961559102e-06, 2.244599219519637e-06, 2.2965480634841707e-06, 2.3977667785381096e-06, 2.174164607300501e-06, 2.7121223641529984e-06, 2.276155401527289e-06, 3.05355310406352e-06, 2.781453743517179e-06, 3.128354597764146e-06, 3.509111752972752e-06, 3.9406700147589e-06, 3.7184481425347605e-06, 4.3437516634229095e-06, 4.425629744962215e-06, 4.5722891773809195e-06, 4.434886140016135e-06, 4.915184548278714e-06, 5.256609677342136e-06, 4.896349918204279e-06, 5.226234053270996e-06, 5.194935429490461e-06, 5.3210090667552654e-06, 5.0763082120449145e-06, 4.96550462597572e-06, 4.634405228331802e-06, 4.973000532057678e-06, 4.286238854928014e-06, 4.697169542742838e-06, 4.509318321887565e-06, 4.201008109152657e-06, 3.858686886247493e-06, 3.7746598916768673e-06, 3.82872204618864e-06, 3.037266603777972e-06, 2.992989598949571e-06, 3.187496020392556e-06, 3.110676723120152e-06, 2.899473680411057e-06, 3.157864215994686e-06, 2.8442307670329785e-06, 3.5490646972872668e-06, 3.3896927850817593e-06, 3.6103464179952295e-06, 3.844670747322278e-06, 3.8027703673424e-06, 4.359131789186167e-06, 4.855231878825097e-06, 5.086570548002924e-06, 5.4424141738427675e-06, 5.573899610739029e-06, 6.457028446883069e-06, 6.558639582030777e-06, 6.682968394132657e-06, 6.7329856150950165e-06, 7.110369478987701e-06, 7.181939523788032e-06, 7.6108852209369375e-06, 7.671224116471207e-06, 8.19534054057914e-06, 8.28518620314012e-06, 8.582277510583474e-06, 8.08159117506255e-06, 8.592771823525195e-06, 8.808623554085261e-06, 8.678481539639976e-06, 8.774782892730746e-06, 8.872867226959289e-06, 9.306989416683405e-06, 8.80079723600486e-06, 8.923316328547296e-06, 8.857316821261158e-06, 8.497018303038633e-06, 8.450302147142801e-06, 8.330103186078004e-06, 8.181589148700388e-06, 8.364640053346024e-06, 8.089522402410945e-06, 8.038486854906784e-06, 7.559377239224447e-06, 7.834472519054424e-06, 7.606287791920612e-06, 7.229592121460503e-06, 6.7413904195003394e-06, 6.673940905367487e-06, 6.502019664253954e-06, 6.11230068050048e-06, 6.186047713195388e-06, 5.512615728158219e-06, 5.56957607803151e-06, 5.391278785837193e-06, 5.201962050114098e-06, 5.122693792590208e-06, 4.884111786112249e-06, 4.561078632495525e-06, 4.348181693355761e-06, 3.873526080571724e-06, 4.127271669892925e-06, 3.621677936450303e-06, 3.4484572462757395e-06, 3.719756611302653e-06, 3.3478386454406027e-06, 3.0847379484905603e-06, 3.3901555584310103e-06, 3.084380463350091e-06, 2.938725624199502e-06, 2.9510121086944756e-06, 2.6612294334413135e-06, 2.878880609389868e-06, 2.9860169933389707e-06, 2.73056278655256e-06, 2.661337385791646e-06, 2.9461387537803366e-06, 2.988087021597346e-06, 2.5218132582104345e-06, 2.8806922036943222e-06, 3.139471660945584e-06, 2.850651154464484e-06, 3.1385559933186773e-06, 3.0390762000802715e-06, 2.827980033546525e-06, 3.1051274215266232e-06, 3.0537590301833586e-06, 3.4067430044164756e-06, 3.1235557742110356e-06, 3.299395637036747e-06, 3.2757864321618387e-06, 3.806191532426912e-06, 3.2709351340655545e-06, 3.553718573973196e-06, 3.826398877873575e-06, 4.005941264806998e-06, 3.8023970432980715e-06, 3.7769031177125618e-06, 4.285766600413342e-06, 4.21567624992605e-06, 4.804269075695291e-06, 4.049224789490171e-06, 4.806103472770055e-06, 4.780636035991207e-06, 4.743774569653859e-06, 4.875745171295571e-06, 5.069980984578401e-06, 5.720287913722799e-06, 5.548710217539509e-06, 5.809313470725494e-06, 5.702497661530186e-06, 6.119268906751704e-06, 6.009344572565215e-06, 6.32930835638014e-06, 6.248462768612534e-06, 6.608800347075161e-06, 6.471897420669416e-06, 6.570502812009838e-06, 6.80090292548595e-06, 6.811388306200372e-06, 7.078605525527552e-06, 7.042635144727451e-06, 7.05281532501396e-06, 7.286601318306631e-06, 7.411755239110693e-06, 6.841280215199346e-06, 7.118682924930314e-06, 7.09661432941185e-06, 7.143397556480814e-06, 7.146454313212496e-06, 7.108018016969385e-06, 7.328632020674906e-06, 7.425015840426838e-06, 7.024449168722821e-06, 7.065751957113601e-06, 6.897643286488025e-06, 6.992318823812692e-06, 6.866747253678889e-06, 6.84686810509781e-06, 6.859506006118252e-06, 6.750332865406658e-06, 6.680754730061978e-06, 6.3020543731669686e-06, 6.387930831054964e-06, 6.360419526955584e-06, 5.984543859018201e-06, 6.233430233494072e-06, 6.109506713043461e-06, 5.972463572598748e-06, 5.980510147354285e-06, 5.81550965815337e-06, 5.530293856344037e-06, 5.490776833215111e-06, 5.49377834896694e-06, 5.557188454582217e-06, 5.491934441354328e-06, 5.361394986998592e-06, 5.084652293129359e-06, 5.110655956270496e-06, 4.585097892400947e-06, 5.082326985437911e-06, 4.637797231892828e-06, 4.7723484855611556e-06, 4.810519551784839e-06, 4.721587743135995e-06, 4.571258783122317e-06, 4.627634458272948e-06, 4.725415982447056e-06, 4.720076107525171e-06, 4.472548094831452e-06, 4.550669868671273e-06]]
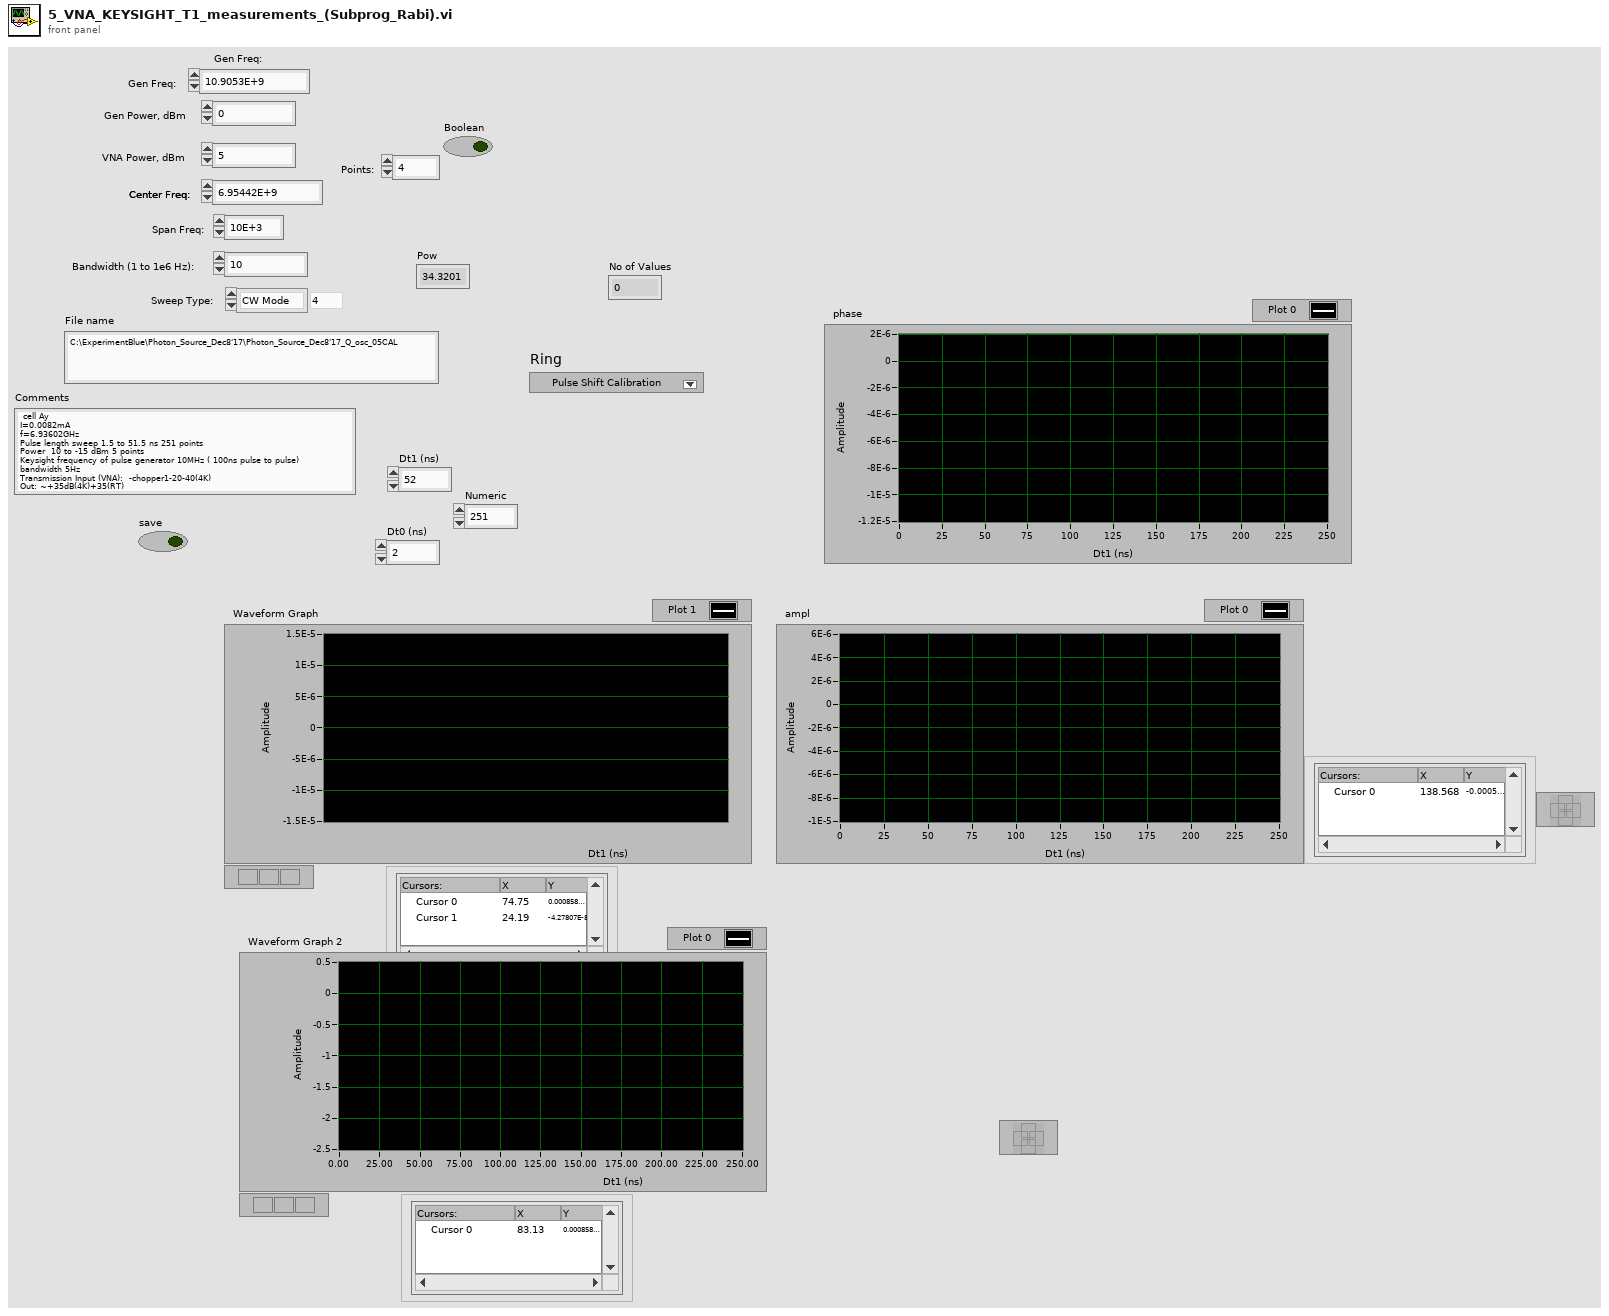
[diagram p1: front panel]
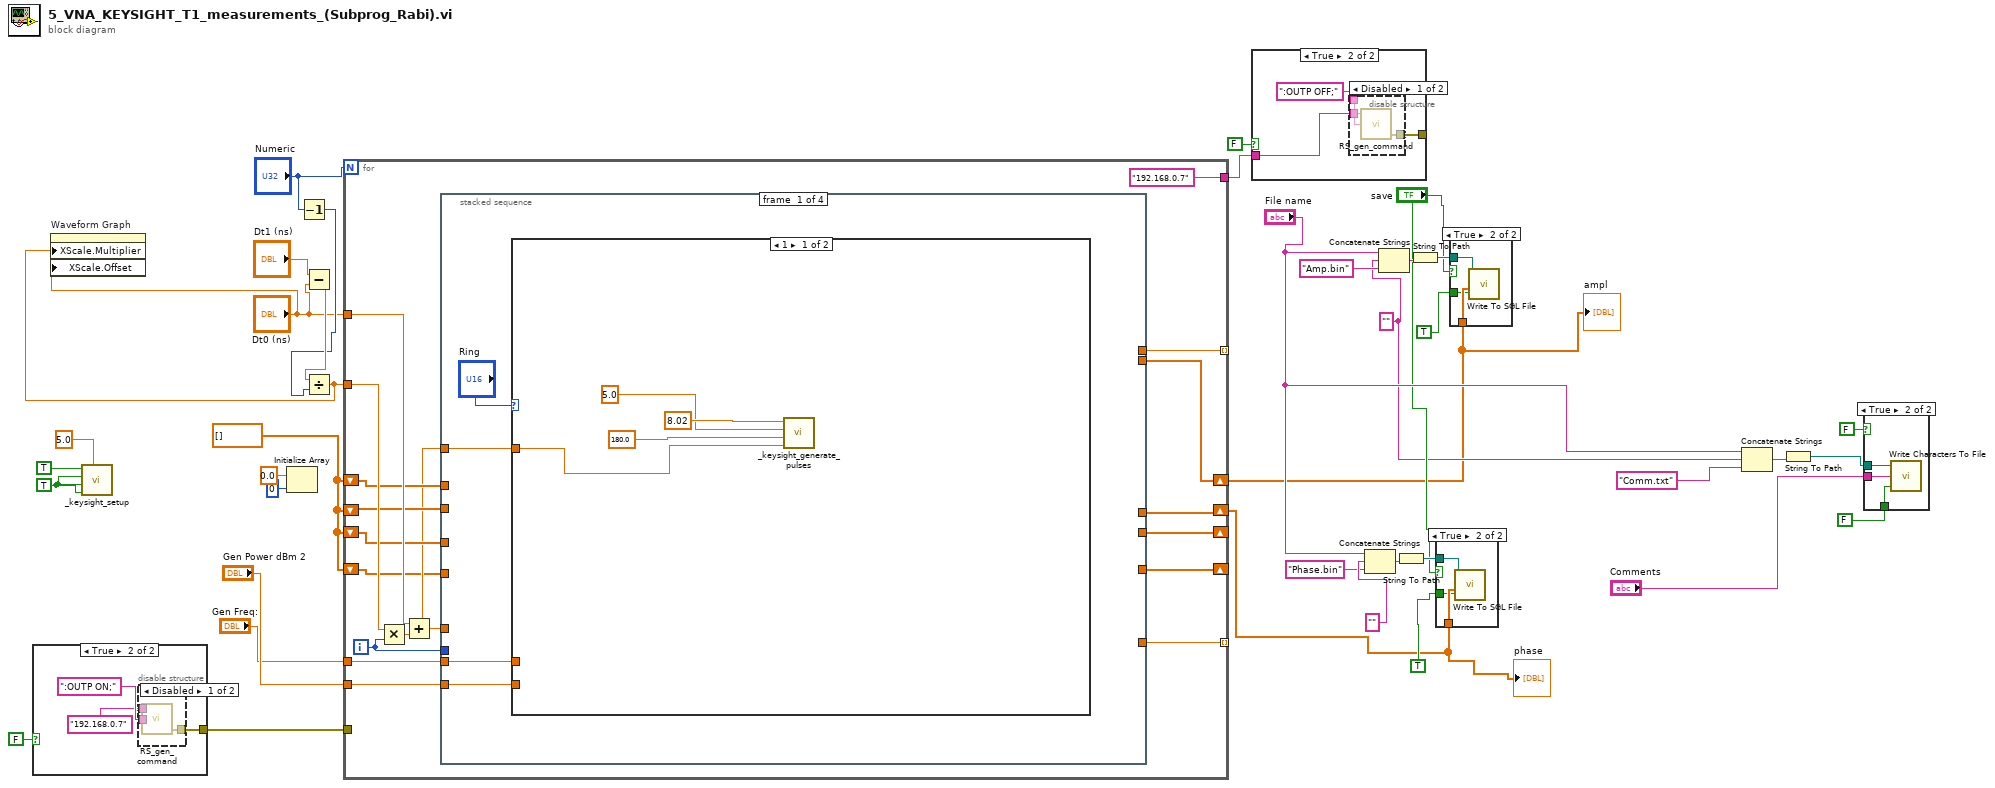
[diagram p0: block diagram]
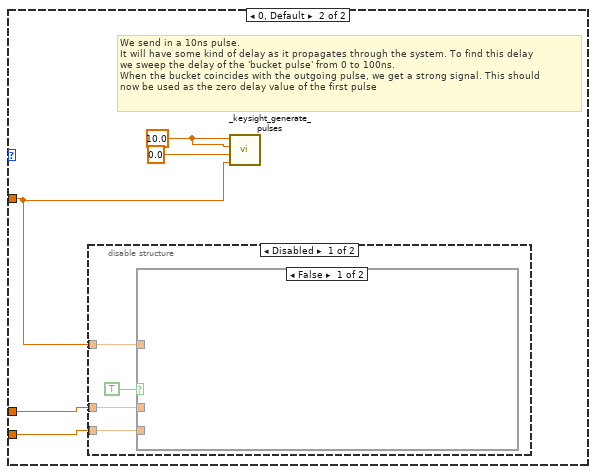
[diagram p9: hidden frame]
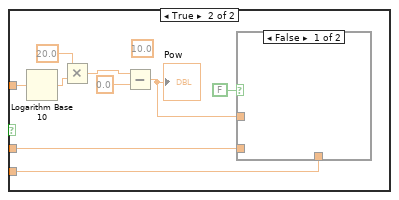
[diagram p10: hidden frame]
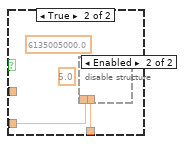
[diagram p11: hidden frame]
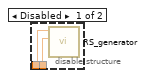
[diagram p12: hidden frame]
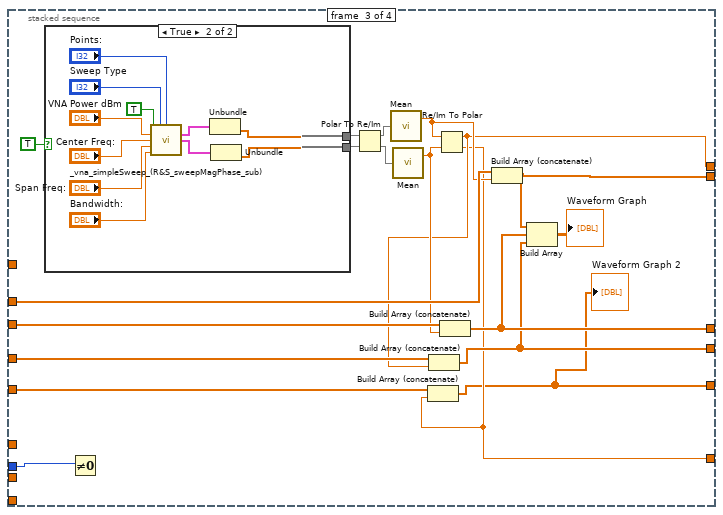
[diagram p15: hidden frame]
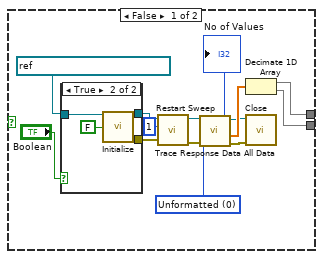
[diagram p16: hidden frame]
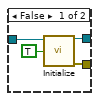
[diagram p17: hidden frame]
diagram:
  w3 = TRUE ("Ouput 1")
  w16 = "" ("format string")
  w6 = dbl[] []
  n1 = case shown="True" FALSE {
    tunnel: [_ w39] -> w11
    frame False {
    }
    frame True {
      n2 = disable-structure shown="Disabled" {
        disable-tunnel: ":OUTP ON;" -> [w44 _]
        disable-tunnel: "192.168.0.7" ("address") -> [w43 _]
        disable-tunnel: [w42 _] -> w39
        frame Disabled {
          n3 = call "RS_gen_command.vi"("Comand"=w44, "address"=w43) -> ("error out"=w42:errorcluster)  [unwired: 3 in]
        }
        frame Enabled {
        }
      }
    }
  }
  n4 = call "_keysight_setup.vi"("Frequency (MHz)"=5.0, "Ouput 2 Neg"=w3, "Ouput 1 Neg"=w3, "Ouput 2"=w3, "Ouput 1"=TRUE) -> ()  [unwired: 1 in, 2 out]
  n5 = Initialize Array(0.0 ("element"), 0 ("dimension size")) -> ()  [unwired: 1 out]
  n6 = Decrement(x="Numeric") -> (x-1=w35:u32)
  n7 = Subtract(x="Dt1 (ns)", y="Dt0 (ns)") -> (x-y=w36:dbl)
  n8 = Divide(x=w36, y=w35) -> (x/y=w1:dbl)
  n9 = property on="Waveform Graph" class="WFGraph (strict)"("XScale.Multiplier"=w1, "XScale.Offset"="Dt0 (ns)") -> ()  [unwired: 2 in, 2 out]
  n10 = for {
    N: "Numeric" -> [_]
    tunnel: w1 -> [w62]
    tunnel: "Dt0 (ns)" -> [w60]
    shift-right: [w58] -> w8
    shift-left: w6 -> [w59]
    shift-right: [w56] -> w7
    shift-left: w6 -> [w57]
    shift-right: [w54] -> _
    shift-left: w6 -> [w53]
    tunnel: "Gen Power dBm 2" -> [w51]
    tunnel: "Gen Freq:" -> [w50]
    tunnel: w11 -> [_]
    tunnel: ["192.168.0.7" ("address")] -> w9
    tunnel: [w48] -> _ mode=indexing
    tunnel: [w47] -> _ mode=indexing
    shift-right: [w45] -> _
    shift-left: w6 -> [w46]
    i -> [w55]
    n11 = Multiply(x=w62, y=w55) -> (x*y=w61:dbl)
    n12 = Add(x=w60, y=w61) -> (x+y=w52:dbl)
    n13 = stacked-sequence {
      tunnel: w52 -> [w66 _ _ _]
      tunnel: w59 -> [_ _ w111 _]
      tunnel: [_ _ w102 _] -> w58
      tunnel: w57 -> [_ _ w106 _]
      tunnel: [_ _ w100 _] -> w56
      tunnel: w55 -> [_ _ w101 _]
      tunnel: [_ _ w98 _] -> w54
      tunnel: w53 -> [_ _ w99 _]
      tunnel: w52 -> [_ _ _ _]
      tunnel: w51 -> [w64 _ _ _]
      tunnel: w50 -> [w63 _ _ _]
      tunnel: [_ _ w96 _] -> w48
      tunnel: [_ _ w94 _] -> w47
      tunnel: w46 -> [_ _ w95 _]
      tunnel: [_ _ w93 _] -> w45
      frame #0 {
        n14 = case shown="1" "Ring" {
          tunnel: w66 -> [w69 w71]
          tunnel: w64 -> [_ w75]
          tunnel: w63 -> [_ w74]
          frame 1 {
            n15 = call "_keysight_generate_pulses.vi"("Ch1 pulse_width (ns)"=8.02, "Ch2 pulse_width (ns)"=5.0, "Ch1 pulse_delay (ns)"=180.0, "Ch2 pulse_delay (ns)"=w69) -> ()  [unwired: 1 in, 2 out]
          }
          frame 0, Default {
            w73 = 10.0 ("Ch1 pulse_width (ns)")
            # "We send in a 10ns pulse.\nIt will have some kind of delay as it propagates through the system. To find this delay\nwe sweep the delay of the 'bucket pulse' from 0 to 100ns. \nWhen the bucket coincides with the outgoing pulse, we get a strong signal. This should\nnow be used as the zero delay value of the first pulse"
            n16 = disable-structure shown="Disabled" {
              disable-tunnel: w75 -> [w78 _]
              disable-tunnel: w74 -> [w77 _]
              disable-tunnel: w71 -> [w76 _]
              frame Disabled {
                n17 = case shown="False" TRUE {
                  tunnel: w76 -> [_ w82]
                  tunnel: w78 -> [_ w81]
                  tunnel: w77 -> [_ w80]
                  frame False {
                  }
                  frame True {
                    (unwired) 10.0
                    n18 = Logarithm Base 10(1:w82) -> (0:w87:dbl)
                    n19 = Multiply(x=20.0, y=w87) -> (x*y=w85:dbl)
                    n20 = Subtract(x=w85, y=0.0) -> (x-y=w83:dbl)
                    "Pow" <- w83
                    n21 = case shown="False" FALSE {
                      tunnel: w83 -> [_ _]
                      tunnel: w81 -> [_ w90]
                      tunnel: w80 -> [_ w89]
                      frame False {
                      }
                      frame True {
                        (unwired) 5.0 ("Power  (dBm)")
                        (unwired) 6135005000.0 ("F (GHz)")
                        n22 = disable-structure shown="Enabled" {
                          disable-tunnel: w90 -> [w92 _]
                          disable-tunnel: w89 -> [w91 _]
                          frame Disabled {
                            n23 = call "RS_generator.vi"("Power  (dBm)"=w92, "Frequency (Hz)"=w91) -> ()  [unwired: 10 in]
                          }
                          frame Enabled {
                          }
                        }
                      }
                    }
                  }
                }
              }
              frame Enabled {
              }
            }
            n24 = call "_keysight_generate_pulses.vi"("Ch1 pulse_width (ns)"=w73, "Ch2 pulse_width (ns)"=w73, "Ch1 pulse_delay (ns)"=0.0, "Ch2 pulse_delay (ns)"=w71) -> ()  [unwired: 1 in, 2 out]
          }
        }
      }
      frame #1 {
      }
      frame #2 {
        n25 = case shown="True" TRUE {
          tunnel: [w119 w134] -> w110
          tunnel: [w118 w135] -> w109
          frame False {
            w124 = 0 items=["Unformatted", "Formatted", "Unformatted With Trace Mathematics"] ("Data Format (Unformatted)")
            n26 = case shown="True" "Boolean" {
              tunnel: [w126 w133] -> w115
              tunnel: [w127 w132] -> w117
              tunnel: refnum<visa-resource-name> "TCPIP::192.168.0.3::INST" ("VISA resource name") -> [w128 w131]
              frame False {
                n27 = call <instrlib>:"Initialize.vi"("VISA resource name"=w128, "Reset (T: Reset)"=TRUE) -> ("VISA resource name out"=w127:refnum<visa-resource-name>, "error out"=w126:errorcluster)  [unwired: 12 in]
              }
              frame True {
                n28 = call <instrlib>:"Initialize.vi"("VISA resource name"=w131, "Reset (T: Reset)"=FALSE) -> ("VISA resource name out"=w132:refnum<visa-resource-name>, "error out"=w133:errorcluster)  [unwired: 12 in]
              }
            }
            n29 = call <instrlib>:"Restart Sweep.vi"("error in (no error)"=w115, "Channel (1)"=1, "VISA resource name"=w117) -> ("error out"=w114:errorcluster, "VISA resource name out"=w116:refnum<visa-resource-name>)  [unwired: 7 in]
            n30 = call <instrlib>:"Trace Response Data All Data.vi"("error in (no error)"=w114, "Data Format (Unformatted)"=w124, "VISA resource name"=w116) -> ("error out"=w123:errorcluster, "Trace Data"=w125:dbl[], "No of Values"=→"No of Values":i32, "VISA resource name out"=w122:refnum<visa-resource-name>)  [unwired: 5 in]
            n31 = Decimate 1D Array(w125) -> (w119:dbl[], w118:dbl[])
            n32 = call <instrlib>:"Close.vi"("error in (no error)"=w123, "VISA resource name"=w122) -> ()  [unwired: 9 in, 1 out]
          }
          frame True {
            n33 = call "_vna_simpleSweep_(R&S_sweepMagPhase_sub).vi"("Boolean"=TRUE, "Sweep Type"="Sweep Type", "Points:"="Points:", "Power dBm"="VNA Power dBm", "Center Freq:"="Center Freq:", "Span Freq:"="Span Freq:", "Bandwidth:"="Bandwidth:") -> ("Lin Mag"=w136:cluster{dbl[], dbl[]}, "Phase"=w137:cluster{dbl[], dbl[]})  [unwired: 7 in]
            n34 = Unbundle(w136) -> (w134:dbl[])  [unwired: 1 out]
            n35 = Unbundle(w137) -> (w135:dbl[])  [unwired: 1 out]
          }
        }
        n36 = Not Equal To 0?(x=w101) -> ()  [unwired: 1 out]
        n37 = Polar To Re/Im(2:w109, 3:w110) -> (0:w107:dbl[], 1:w108:dbl[])
        n38 = call-poly <vilib>:"Mean.vi"("X"=w108) -> ("mean"=w104:dbl)  [unwired: 1 out]
        n39 = call-poly <vilib>:"Mean.vi"("X"=w107) -> ("mean"=w105:dbl)  [unwired: 1 out]
        n40 = Re/Im To Polar(2:w105, 3:w104) -> (0:w94:dbl, 1:w96:dbl)
        n41 = Build Array (concatenate)(w95, w94) -> (w93:dbl[])
        "Waveform Graph 2" <- w93
        n42 = Build Array (concatenate)(w99, w96) -> (w98:dbl[])
        n43 = Build Array (concatenate)(w106, w105) -> (w100:dbl[])
        n44 = Build Array (concatenate)(w111, w104) -> (w102:dbl[])
        n45 = Build Array(w102, w100, w98) -> (→"Waveform Graph":dbl[][])
      }
      frame #3 {
      }
    }
  }
  "ampl" <- w8
  "phase" <- w7
  n46 = case shown="True" FALSE {
    tunnel: [_ w146] -> _
    tunnel: w9 -> [_ w145]
    frame False {
    }
    frame True {
      n47 = disable-structure shown="Disabled" {
        disable-tunnel: ":OUTP OFF;" -> [w150 _]
        disable-tunnel: [w149 _] -> w146
        disable-tunnel: w145 -> [w148 _]
        frame Disabled {
          n48 = call "RS_gen_command.vi"("Comand"=w150, "address"=w148) -> ("error out"=w149:errorcluster)  [unwired: 3 in]
        }
        frame Enabled {
        }
      }
    }
  }
  n49 = Concatenate Strings("File name", "" ("format string"), "Phase.bin") -> (w26:string)
  n50 = Concatenate Strings("File name", w16, "Amp.bin") -> (w30:string)
  n51 = String To Path(string=w26) -> (path=w28:path)
  n52 = String To Path(string=w30) -> (path=w32:path)
  n53 = case shown="True" "save" {
    tunnel: w28 -> [_ w153]
    tunnel: w7 -> [_ w152]
    tunnel: TRUE -> [_ w151]
    frame False {
    }
    frame True {
      n54 = call <vilib>:"Write To SGL File.vi"("append to file? (new file:F)"=w151, "1D array"=w152, "file path (dialog if empty)"=w153) -> ()  [unwired: 4 in, 1 out]
    }
  }
  n55 = case shown="True" "save" {
    tunnel: w32 -> [_ w156]
    tunnel: w8 -> [_ w155]
    tunnel: TRUE -> [_ w154]
    frame False {
    }
    frame True {
      n56 = call <vilib>:"Write To SGL File.vi"("append to file? (new file:F)"=w154, "1D array"=w155, "file path (dialog if empty)"=w156) -> ()  [unwired: 4 in, 1 out]
    }
  }
  n57 = Concatenate Strings("File name", w16, "Comm.txt") -> (w23:string)
  n58 = String To Path(string=w23) -> (path=w20:path)
  n59 = case shown="True" FALSE {
    tunnel: w20 -> [_ w159]
    tunnel: "Comments" -> [_ w158]
    tunnel: FALSE -> [_ w157]
    frame False {
    }
    frame True {
      n60 = call <vilib>:"Write Characters To File.vi"("append to file? (new file:F)"=w157, "character string"=w158, "file path (dialog if empty)"=w159) -> ()  [unwired: 2 in, 1 out]
    }
  }
